vi "Camera_Crop_X_Axis.vi"(9 "Detect Movement":bool, 10 "Camera":T1, 11 "input cluster":T2={"Pinch-valve"="", "XLP 6000 Pump"="", "Camera1"="", "Camera2"="", "Img_Capt"=FALSE, "Actuator"=FALSE, "Pump"=FALSE, "Cam 1"=FALSE, "Cam 2"=FALSE, "Empty_Refill"=FALSE, "Crop"=FALSE, "Light intensity"=0, "Exposure Time"=0.0, "Sample Name"="", "Operator"="", "Calibration 1"=path "", "Calibration 2"=path "", "Framerate"=0, "Timeout Sample"=0, "Collection date"="", "Sample size threshold"=0, "Empty start"=0, "Command"="", "Station"="", "Species Name"="", "Other Notes"="", "Aperture"=enum."Item 0", "Image Process Queue Size"=0, "Image Save Queue Size"=0, "Overload threshold"=0, "Max Framerate"=0, "Rectangle 1"={"Left"=0, "Top"=0, "Right"=0, "Bottom"=0, "Rotation"=0.0}, "Rectangle 2"={"Left"=0, "Top"=0, "Right"=0, "Bottom"=0, "Rotation"=0.0}, "Detection Region %"=200.0, "Detect 1"=path "", "Detect 2"=path "", "Max large object threshold"=500, "Open(T)/Close(F)"=FALSE, "Img_Capt Begin"=FALSE, "Dispense Speed"=0, "Flush Size"=0, "Location"="", "Latitude"="", "Longitude"="", "Determiner"="", "Sex"="", "Camera1_Img"=refnum, "Camera2_Img"=refnum, "Img1_Orig_Disp"=refnum, "Img2_Orig_Disp"=refnum, "Img1_Orig_RGB"=refnum, "Img2_Orig_RGB"=refnum, "Blue_Plane_Extract"=refnum, "Subtracted_Plane"=refnum, "Img1_Binary"=refnum, "Img2_Binary"=refnum, "Crop_Mask"=refnum, "Img1_Save"=refnum, "Img2_Save"=refnum, "Img1_Cali_Full"=refnum, "Img2_Cali_Full"=refnum, "Img1_Cali_Detect"=refnum, "Img2_Cali_Detect"=refnum, "Cam 1 queue"=refnum, "Cam 2 queue"=refnum, "Cam 1 - save queue"=refnum, "Cam 2 - save queue"=refnum, "Overlay_Ring"=0, "SystemVersion"=0, "System Serial"="", "Legacy Cam Attributes"=FALSE, "Camera Orientation 1"="", "Camera Orientation 2"="", "Pixel to mm 1"=0.0, "Pixel to mm 2"=0.0, "CAM1 Model"=enum."a2A5328-15ucBAS", "CAM2 Model"=enum."a2A5328-15ucBAS", "Flush Insect"=FALSE, "Pump Size"=FALSE, "Barcode"="", "Phase3"=FALSE, "Mega F3"="", "Container nr."=0.0, "Mannual F3"=TRUE} {"SystemVersion" items=["Standard", "XL"]; "Overlay_Ring" items=["Session Data", "Extended Setup", "Buffer", "Camera", "Dispenser", "Stats", "Connections"]; "Flush Size" min=1; "Dispense Speed" min=1; "Rectangle 2"."Rotation" format="%.2f"; "Rectangle 2"."Left" scale=0.0..1024.0; "Rectangle 2"."Right" scale=0.0..1024.0; "Rectangle 1"."Rotation" format="%.2f"; "Rectangle 1"."Left" scale=0.0..1024.0; "Rectangle 1"."Right" scale=0.0..1024.0; "Max Framerate" min=1; "Overload threshold" min=1; "Image Save Queue Size" min=1; "Image Process Queue Size" min=1; "Empty start" min=1; "Sample size threshold" min=1; "Framerate" min=1; "Light intensity" scale=0.0..100.0}) -> (1 "Width":i64, 3 "OffsetX":i64)   [LabVIEW 2024]
uses:
  controls/Data.ctl
  <vilib>/userDefined/High Color/IMAQdx.ctl
  <vilib>/vision/Image Controls.llb/IMAQ Image.ctl
  Camera_ID.ctl
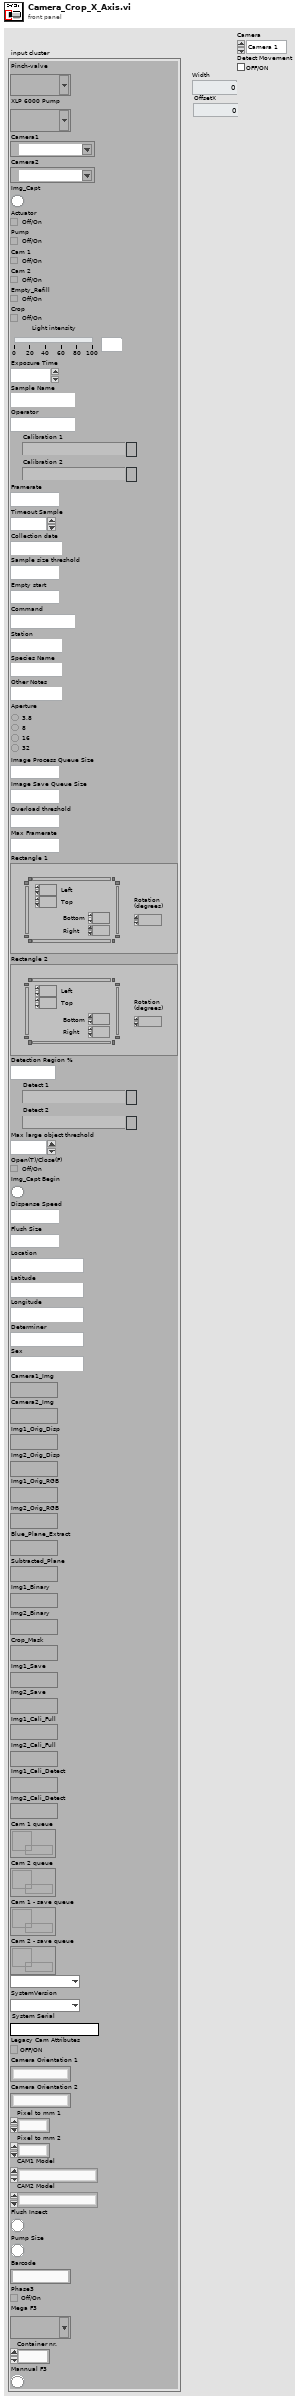
[diagram p1: front panel]
types:
  T1 = typedef "Camera_ID.ctl" = enum16{"Camera 1", "Camera 2"}
  T2 = typedef "Data.ctl" = cluster{"Pinch-valve":refnum<visa-resource-name>, "XLP 6000 Pump":refnum<visa-resource-name>, "Camera1":T3, "Camera2":T3, "Img_Capt":bool, "Actuator":bool, "Pump":bool, "Cam 1":bool, "Cam 2":bool, "Empty_Refill":bool, "Crop":bool, "Light intensity":i32, "Exposure Time":dbl, "Sample Name":string, "Operator":string, "Calibration 1":path, "Calibration 2":path, "Framerate":i32, "Timeout Sample":i32, "Collection date":string, "Sample size threshold":i32, "Empty start":u32, "Command":string, "Station":string, "Species Name":string, "Other Notes":string, "Aperture":enum32{"Item 0", "Item 1", "Item 2", "Item 3"}, "Image Process Queue Size":i32, "Image Save Queue Size":i32, "Overload threshold":i32, "Max Framerate":i32, "Rectangle 1":T4, "Rectangle 2":T4, "Detection Region %":dbl, "Detect 1":path, "Detect 2":path, "Max large object threshold":i32, "Open(T)/Close(F)":bool, "Img_Capt Begin":bool, "Dispense Speed":i32, "Flush Size":i32, "Location":string, "Latitude":string, "Longitude":string, "Determiner":string, "Sex":string, "Camera1_Img":T5, "Camera2_Img":T5, "Img1_Orig_Disp":T5, "Img2_Orig_Disp":T5, "Img1_Orig_RGB":T5, "Img2_Orig_RGB":T5, "Blue_Plane_Extract":T5, "Subtracted_Plane":T5, "Img1_Binary":T5, "Img2_Binary":T5, "Crop_Mask":T5, "Img1_Save":T5, "Img2_Save":T5, "Img1_Cali_Full":T5, "Img2_Cali_Full":T5, "Img1_Cali_Detect":T5, "Img2_Cali_Detect":T5, "Cam 1 queue":refnum<queue>, "Cam 2 queue":refnum<queue>, "Cam 1 - save queue":refnum<queue>, "Cam 2 - save queue":refnum<queue>, "Overlay_Ring":u16, "SystemVersion":u16, "System Serial":string, "Legacy Cam Attributes":bool, "Camera Orientation 1":string, "Camera Orientation 2":string, "Pixel to mm 1":dbl, "Pixel to mm 2":dbl, "CAM1 Model":enum16{"a2A5328-15ucBAS", "acA1920-155uc"}, "CAM2 Model":enum16{"a2A5328-15ucBAS", "acA1920-155uc"}, "Flush Insect":bool, "Pump Size":bool, "Barcode":string, "Phase3":bool, "Mega F3":refnum<visa-resource-name>, "Container nr.":dbl, "Mannual F3":bool}
  T3 = typedef "IMAQdx.ctl" = refnum<k21>
  T4 = typedef "IMAQ Rectangle" = cluster{"Left":i32, "Top":i32, "Right":i32, "Bottom":i32, "Rotation":dbl}
  T5 = typedef "IMAQ Image.ctl" = refnum<image>
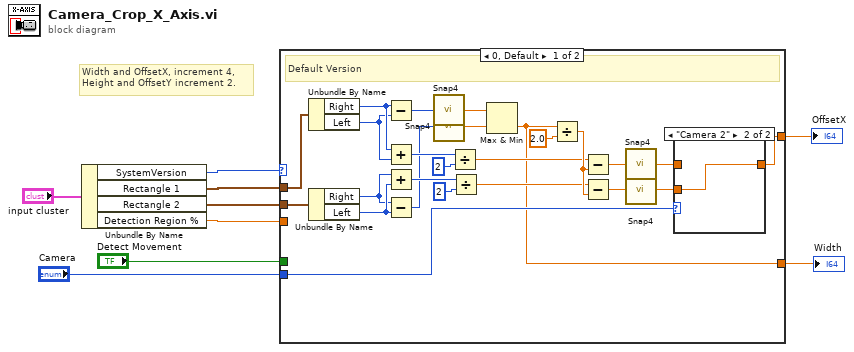
[diagram p0: block diagram]
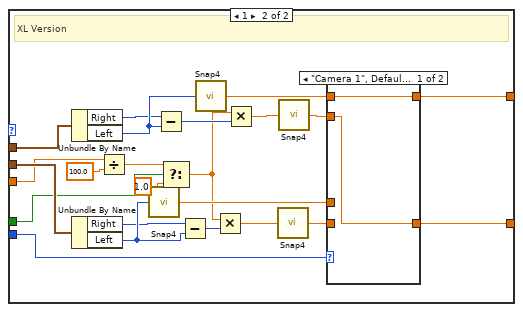
[diagram p3: hidden frame]
diagram:
  # "Width and OffsetX, increment 4,\nHeight and OffsetY increment 2."
  n1 = Unbundle By Name("input cluster") -> ("SystemVersion"=w5:u16, "Rectangle 1"=w7:T4, "Rectangle 2"=w8:T4, "Detection Region %"=w4:dbl)
  n2 = case shown="0, Default" w5 {
    tunnel: w8 -> [w30 w53]
    tunnel: w7 -> [w24 w54]
    tunnel: "Camera" -> [w22 w50]
    tunnel: [w14 w48] -> w1
    tunnel: [w19 w49] -> w2
    tunnel: w4 -> [_ w52]
    tunnel: "Detect Movement" -> [_ w51]
    frame 0, Default {
      # "Default Version"
      n3 = Unbundle By Name(w24) -> ("Right"=w16:i32, "Left"=w15:i32)
      n4 = Unbundle By Name(w30) -> ("Right"=w17:i32, "Left"=w18:i32)
      n5 = Subtract(x=w16, y=w15) -> (x-y=w10:i32)
      n6 = Add(x=w16, y=w15) -> (x+y=w25:i32)
      n7 = Add(x=w17, y=w18) -> (x+y=w28:i32)
      n8 = Subtract(x=w17, y=w18) -> (x-y=w13:i32)
      n9 = call "Snap4.vi"("x"=w10) -> ("x out"=w11:dbl)
      n10 = call "Snap4.vi"("x"=w13) -> ("x out"=w12:dbl)
      n11 = Divide(x=w25, y=2) -> (x/y=w27:dbl)
      n12 = Divide(x=w28, y=2) -> (x/y=w31:dbl)
      n13 = Max & Min(x=w11, y=w12) -> (min(x,y)=w14:dbl)  [unwired: 1 out]
      n14 = Divide(x=w14, y=2.0) -> (x/y=w32:dbl)
      n15 = Subtract(x=w27, y=w32) -> (x-y=w33:dbl)
      n16 = Subtract(x=w31, y=w32) -> (x-y=w34:dbl)
      n17 = call "Snap4.vi"("x"=w33) -> ("x out"=w21:dbl)
      n18 = call "Snap4.vi"("x"=w34) -> ("x out"=w20:dbl)
      n19 = case shown="\"Camera 2\"" w22 {
        tunnel: w21 -> [w35 _]
        tunnel: [w35 w36] -> w19
        tunnel: w20 -> [_ w36]
        frame "Camera 1", Default {
        }
        frame "Camera 2" {
        }
      }
    }
    frame 1 {
      # "XL Version"
      n20 = Unbundle By Name(w54) -> ("Right"=w40:i32, "Left"=w47:i32)
      n21 = Unbundle By Name(w53) -> ("Right"=w41:i32, "Left"=w46:i32)
      n22 = Divide(x=w52, y=100.0 ("x")) -> (x/y=w58:dbl)
      n23 = call "Snap4.vi"("x"=w46) -> ("x out"=w56:dbl)
      n24 = Subtract(x=w40, y=w47) -> (x-y=w45:i32)
      n25 = Select(t=w58, s=w51, f=1.0 ("t")) -> (s? t:f=w37:dbl)
      n26 = Subtract(x=w41, y=w46) -> (x-y=w43:i32)
      n27 = call "Snap4.vi"("x"=w47) -> ("x out"=w55:dbl)
      n28 = Multiply(x=w37, y=w43) -> (x*y=w38:dbl)
      n29 = Multiply(x=w37, y=w45) -> (x*y=w39:dbl)
      n30 = call "Snap4.vi"("x"=w38) -> ("x out"=w42:dbl)
      n31 = call "Snap4.vi"("x"=w39) -> ("x out"=w44:dbl)
      n32 = case shown="\"Camera 1\", Default" w50 {
        tunnel: w56 -> [_ w63]
        tunnel: [w61 w63] -> w49
        tunnel: w44 -> [w60 _]
        tunnel: [w60 w62] -> w48
        tunnel: w55 -> [w61 _]
        tunnel: w42 -> [_ w62]
        frame "Camera 1", Default {
        }
        frame "Camera 2" {
        }
      }
    }
  }
  "Width" <- w1
  "OffsetX" <- w2
